vi "Savitzky-Golay Filter.vi"   [LabVIEW 2010, in "NI_AALBase.lvlib"]
doc: "Filters the input data sequence<B> X</B> using a Savitzky-Golay FIR smoothing filter. Wire data to the <B>X</B> input to determine the polymorphic instance to use or manually select the instance."
uses:
  NI_AALBase.lvlib
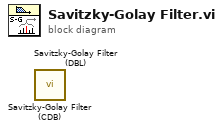
[diagram p0: block diagram]
diagram:
  n1 = call "Savitzky-Golay Filter (CDB).vi"() -> ()  [unwired: 10 in, 2 out]
  n2 = call "Savitzky-Golay Filter (DBL).vi"() -> ()  [unwired: 10 in, 2 out]
